vi "Global_Read.vi"() -> ()   [LabVIEW 2011]
panel:
  in  "Global Read":bool
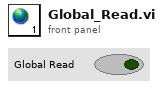
[diagram p1: front panel]
diagram:
